vi "StartLoggingChannels.vi"(8 "error in (no error)":errorcluster, 9 "Data Log File Configuration":T1={"File Path"=path "", "Description"="", "Trigger"={"Type"=enum."None", "Channel Path"="", "High Limit"=0.0, "Low Limit"=0.0}, "Replace File"=FALSE, "Rate [Hz]"=1.0, "File Properties"=[], "Channels"=[]}, 10 "Data Log Configuration Name":string="Log", 11 "VeriStand Test Case in":refnum<class "VeriStandTestCase.lvclass">) -> (0 "error out":errorcluster, 3 "VeriStand Test Case out":refnum<class "VeriStandTestCase.lvclass">)   [LabVIEW 2015, in "VeriStandTestCase.lvclass"]
uses:
  VeriStandTestCase.lvclass
  <vilib>/NI Veristand/Execution/Workspace/LogFileConfiguration.ctl
  <vilib>/NI Veristand/Execution/Workspace/LogFileTriggerConfiguration.ctl
  <vilib>/NI Veristand/Execution/Workspace/LogFileTriggerType.ctl
  <vilib>/NI Veristand/Execution/Workspace/LogProperty.ctl
  <vilib>/NI Veristand/Execution/Workspace/LogChannelConfiguration.ctl
  VeriStandTestCase.lvclass/VeriStandTestCase.ctl
  <vilib>/NI VeriStand/Execution/Workspace/NI_VS Workspace ExecutionAPI.lvlib
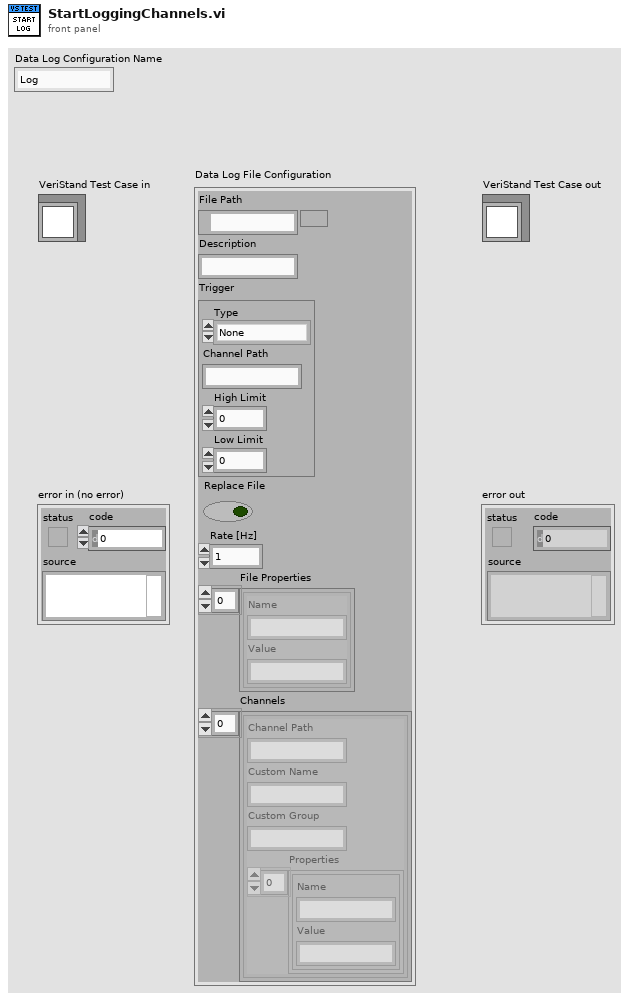
[diagram p1: front panel]
types:
  T1 = typedef "NI_VS Workspace ExecutionAPI.lvlib/LogFileConfiguration.ctl" = cluster{"File Path":path, "Description":string, "Trigger":T2, "Replace File":bool, "Rate [Hz]":dbl, "File Properties":T4[], "Channels":T5[]}
  T2 = typedef "NI_VS Workspace ExecutionAPI.lvlib/LogFileTriggerConfiguration.ctl" = cluster{"Type":T3, "Channel Path":string, "High Limit":dbl, "Low Limit":dbl}
  T3 = typedef "NI_VS Workspace ExecutionAPI.lvlib/LogFileTriggerType.ctl" = enum16{"None", "In Limits", "Out of Limits"}
  T4 = typedef "NI_VS Workspace ExecutionAPI.lvlib/LogProperty.ctl" = cluster{"Name":string, "Value":string}
  T5 = typedef "NI_VS Workspace ExecutionAPI.lvlib/LogChannelConfiguration.ctl" = cluster{"Channel Path":string, "Custom Name":string, "Custom Group":string, "Properties":T4[]}
  T6 = typedef "NI_VS Workspace ExecutionAPI.lvlib/WorkspaceAPI.ctl" = refnum<k24>
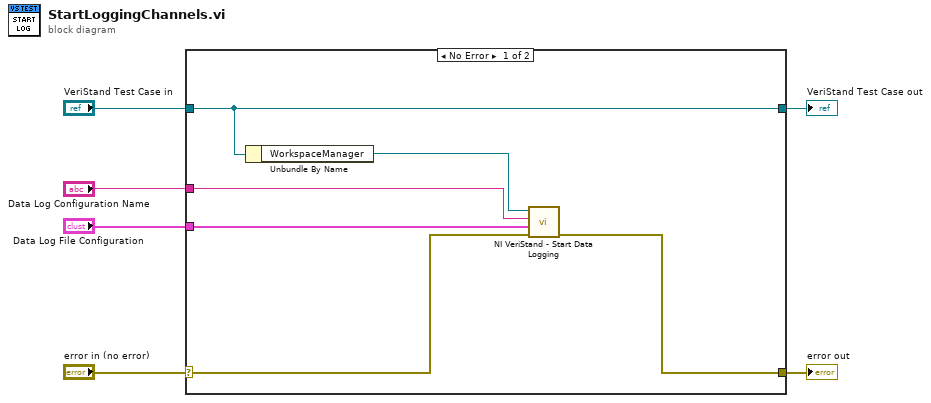
[diagram p0: block diagram]
diagram:
  n1 = case shown="No Error" "error in (no error)" {
    selector: "error in (no error)" -> [w11 w14]
    tunnel: [w10 w14] -> w5
    tunnel: [w9 w13] -> w3
    tunnel: "VeriStand Test Case in" -> [w9 w13]
    tunnel: "Data Log File Configuration" -> [w12 _]
    tunnel: "Data Log Configuration Name" -> [w7 _]
    frame No Error {
      n2 = Unbundle By Name(w9) -> ("WorkspaceManager"=w8:T6)
      n3 = call <vilib>:"NI VeriStand - Start Data Logging.vi"("error in (no error)"=w11, "Data Log File Configuration"=w12, "Data Log Configuration Name"=w7, "WorkspaceManager in"=w8) -> ("error out"=w10:errorcluster)  [unwired: 6 in, 1 out]
    }
    frame Error {
    }
  }
  "error out" <- w5
  "VeriStand Test Case out" <- w3
